vi "Ready.vi"(8 "error in (no error)":errorcluster, 11 "Handle":i16) -> (0 "error out":errorcluster, 2 "x != 0?":bool, 3 "return type":i16)   [LabVIEW 2023]
uses:
  ps2000.dll
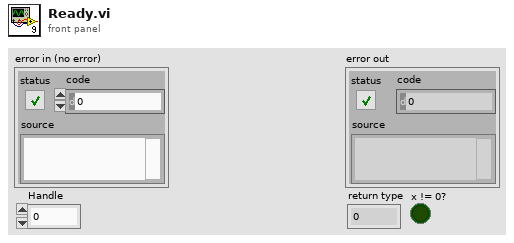
[diagram p1: front panel]
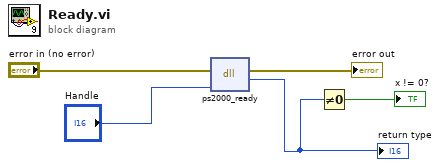
[diagram p0: block diagram]
diagram:
  n1 = dll-call lib="C:/Users/cesar/Desktop/Ps2000 libreria/PS2000.dll" fn="ps2000_ready"(error in="error in (no error)", "Handle"="Handle") -> (error out=→"error out":errorcluster, "return type"=w1:i16)  [unwired: 3 in, 1 out]
  "return type" <- w1
  n2 = Not Equal To 0?(x=w1) -> (x != 0?=→"x != 0?":bool)
